vi "Read Paths to Music Libraries Plugins.vi"(8 "error in (no error)":errorcluster) -> (0 "error out":errorcluster, 3 "Supported Music Libraries":path[](array[path]))   [LabVIEW 2015, in "App Config.lvlib"]
uses:
  App Config.lvlib
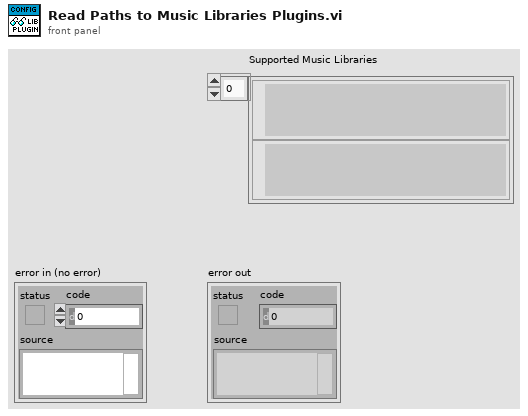
[diagram p1: front panel]
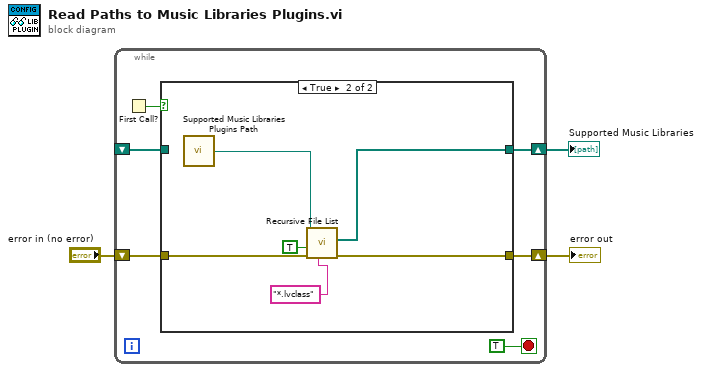
[diagram p0: block diagram]
diagram:
  n1 = while {
    shift-right: [w8] -> w2
    shift-left: "error in (no error)" -> [w9]
    shift-right: [w7] -> w1
    shift-left: _ -> [w4]
    stop <- TRUE stop-if-true
    n2 = First Call?() -> (First Call?: T/F=w6:bool)
    n3 = case shown="True" w6 {
      tunnel: [w11 w12] -> w8
      tunnel: [w10 w13] -> w7
      tunnel: w9 -> [w11 w16]
      tunnel: w4 -> [w10 _]
      frame False {
      }
      frame True {
        n4 = call "Supported Music Libraries Plugins Path.vi"() -> ("Supported Music Libraries Plugins Path"=w15:path)  [unwired: 5 in]
        n5 = call <vilib>:"Recursive File List.vi"("pattern"="*.lvclass" ("regular expression"), "error in (no error)"=w16, "Continue Recursing on Error? (F)"=TRUE, "Folder Path"=w15) -> ("error out"=w12:errorcluster, "All Files in Dir"=w13:path[])  [unwired: 3 in, 3 out]
      }
    }
  }
  "error out" <- w2
  "Supported Music Libraries" <- w1
